vi "Dashboard Main.vi"() -> ()   [LabVIEW 2013]
uses:
  subStates.ctl
  drive safety.ctl
  test controls.ctl
  misc dash data.ctl
  dashboard safety status data.ctl
  <vilib>/event_ctls.llb/lveventtype.ctl
  <vilib>/event_ctls.llb/eventvkey.ctl
  dash error type def.ctl
  <vilib>/Rock Robotics/WPI/DriverStation/WPI_DriverStationDigitalData.ctl
  <vilib>/Utility/config.llb/Write Key (String).vi
  <vilib>/Utility/config.llb/Write Key (I32).vi
  <vilib>/Utility/config.llb/NI_LVConfig.lvlib
panel:
  out "code version":cluster{"code version":string}
  out "connected":string="Connected to robot at IP Address: x.x.x.x"
  in  "Warning No Code":cluster{"Dismiss warning":bool}
  in  "help":bool
  out "no comms":string="NO ROBOT COMMUNICATION"
  in  "no code help":bool
  out "no code":string="NO ROBOT CODE          "
  in  "Warning No Comms":cluster{"Dismiss warning":bool}
  out "Time":string
  out "Drive Safety Data":T1
  out "ip":string="10.0.0.2"
  out "Main Dash SPI":u32
  out "Main Dash IPS":dbl
  out "testmode":bool
  out "lightsense":bool
  out "down":bool
  out "up":bool
  out "unlatched":bool
  out "shooter retracted":bool
  out "Image Message":string="Timeout in Camera Communications"
  in  "Dashboard Tab":T2(tab)
  out "code too slow":bool caption="Robot Code\nRunning too Slow"
  out "Robot Found":bool
  out "BATT":dbl(slide)=12.0 scale=0.0..14.0
  in  "menu":bool
  out "quick data":T4={"Shooter Down"=FALSE, "Shooter Up"=TRUE, "Light Sensor"=FALSE, "Unlatched"=TRUE, "Latched"=TRUE, "State Machine Master"=enum."null", "Dash IPS"=0.0, "Dash mSPI"=0, "Robot IP"="0.0.0.0", "Battery"=16711680, "Code IPS"=0.0, "Code mSPI"=0}
  out "no rate":bool
  out "dist limit":bool
  out "hold":bool
  out "shoot?":bool
  out "Shifter":bool
  out "Vision State":bool
  in  "Camera Settings":T5={"Frame Rate"=30, "Compression"=30, "Size"=1} {"Frame Rate" scale=1.0..30.0; "Size" items=["640x480", "320x240", "160x120"]}
  out "Mode":T6(ring)=enum."Auto Disabled"
  out "Camera IP":string
  in  "DB Camera Config":bool
  out "fps":dbl format="%#.1g"
  out "Mbps":dbl format="%#.1g"
  out "Mbps 2":bool
  out "Distance From Target":dbl
  out "Hot Goal Detected":bool
  out "encoder failure":bool
  out "Directional Failure":bool
  out "TeleOp Elapsed Seconds":dbl
  out "Compressor":u32(colorbox)
  out "info":string="Robot is  in Teleop Disabled"
  out "test disabled":string="Robot is not in Test Mode"
  out "On/Off":bool=TRUE
  out "Full":bool
  out "Charging":bool
  in  "Compressor":bool=TRUE
  out "check settings":string="Check Settings\n\nIf you are trying to test from here,\nchange test mode to dashboard."
  in  "Reset\nManual\nOverrides":bool
  in  "Test \nControls":T7
  out "Test \nIndicators":T8={"Right Distance"=0.0, "Right Rate"=0.0, "Left Distance"=0.0, "Left Rate"=0.0, "Retracted"=TRUE, "Extended"=FALSE, "Shifted Low"=TRUE, "Shifted High"=FALSE, "Unlatched"=TRUE, "Latched"=FALSE, "Directional Issue"=FALSE, "No Rate Read"=FALSE, "Encoder Failure"=FALSE, "At Distance Limit"=FALSE, "Shooter Down"=FALSE, "Shooter Up"=TRUE, "Light Sensor"=FALSE, "Rate"=0.0, "Distance"=0.0, "Right No Rate Read"=FALSE, "Right Encoder Fail"=FALSE, "Left No Rate Read"=FALSE, "LeftEncoder Fail"=FALSE}
  in  "Manual \nOverrides":T9 {"Belts" scale=-1.0..1.0; "Arm" scale=-1.0..1.0; "Drive Train" scale=-1.0..1.0}
  out "timeout error":bool
  out "# of Timeouts":u32
  out "Robot IP\nAddress":string="0.0.0.0"
  out "Solenoid Output":bool[](array[boolean])
  out "8 -- Battery":sgl(graph)
  out "Analog Input":sgl[](array[slide]) scale=0.0..5.0
  out "Drive Encoders":T10
  out "Arm Encoder":cluster{"Distance ":dbl, "Rate":dbl}
  out "Pneumatics":T3
  out "Pickup Arm":T3
  out "Belts":T3
  out "State Machine Master":T3
  out "Drive":T3
  out "Belt Status":u16(ring) items=["Code Control", "Driver Control", "Manual Override"]
  out "Arm Status":u16(ring) items=["Code Control", "Driver Control", "Manual Override"]
  out "Belts":dbl
  out "PWM":cluster{u8, u8}[](array[slide])=[{0, 157}, {0, 157}, {0, 157}, {0, 157}, {0, 157}, {0, 157}, {0, 157}, {0, 157}, {0, 157}, {0, 155}] scale=1.0..255.0
  out "GPIO Output Enable":bool[](array[boolean])
  out "GPIO State":bool[](array[boolean])
  out "Relay":cluster{"Forward":bool[], "Reverse":bool[]}
  out "drive encoder failure":bool
  in  "export stat":bool
  out "Vision mSPI":u32(knob)=100 scale=50.0..200.0
  out "Main mSPI":u32(knob)=20 scale=10.0..40.0
  out "Stats":dbl[][](graph)
  out "cRIO CPU Usage":dbl(knob) scale=0.0..100.0
  out "Vision mSPI":u32
  out "Main mSPI":u32
  out "Main IPS":dbl=50.0
  out "Vision IPS":dbl=10.0
  in  "clear stat":bool
  in  "clear batt":bool
  in  "export batt":bool
  in  "reset":bool
  out "Maximum Voltage":sgl format="%#_gv"
  out "Minimum Voltage":sgl format="%#_gv"
  out "Current Voltage":sgl format="%#_gv"
  out "Battery Stats":sgl(graph)
  in  "Poll Rate (ms)":u32=500
  in  "Listbox":i32(listbox)
  out "Tree":string(tree)
  out "FDC ON":bool
  out "FDC OFF":bool
  in  "Enable Full Driver Control":bool caption="Enables controls with automated functions. Not recommended, since\nthe automated functions were never perfected and are unreliable."
  out "Disable Vision_Off":bool
  out "Disable Vision_On":bool
  in  "Disable Vison After Auto":bool=TRUE caption="After autonomous, vision will be disabled.\nLeave off during practice so multiple \nautonomouses can be run without robot \nreboot being needed. MUST BE ON DURING\nCOMPETITION (DEFAULT)."
  out "Code Version":string
  out "About Speeds":string="Optimal Speeds\n\nMain mSPI = 20\nMain IPS = 50\n\nVision mSPI = 100\nVision IPS = 10\n\nmSPI - miliseconds per iteration\nIPS - iterations per second"
  out "Shoot During\nAuto_Off":bool
  out "Use Hot Goal_Off":bool
  out "2 Ball Auto_Off":bool=TRUE
  out "Shoot During\nAuto_On":bool
  out "Use Hot Goal_On":bool
  out "2 Ball Auto_On":bool
  in  "Shoot During Auto":bool=TRUE caption="When on, shooting sequence will run, \notherwise the robot will just drive forward."
  in  "Use Hot Goal":bool=TRUE caption="Check if the goal is hot when determining \nwhen to shoot, otherwise shoot second cycle."
  in  "2 Ball Auto (Disabled)":bool
  in  "Test Mode":T11(radio)
  in  "Enable":bool
  # "Notification"
  # "!"
  # "C"
  # "No Code"
  # "No robot code has been detected. This means that the code has not \nbegun running yet or there is no code to run.  The code has not\ndeclared to the driver station the code version, so it is assumed \nno code is running."
  # "!"
  # "Warning!"
  # "No robot communication is detected! What to do?\n\n- Is the robot ready and booted? (Blinking RSL)\n- Check robot power.\n- Check various ethernet wire connections on robot and driver station.\n- Check radio power.\n- Robot radio should be on Bridge mode.\n- Check driver station IP address, should be 10.11.24.5, to get it there, simply go to Setup > Choose NIC > Ok (use this espically \n  during competitions). The actual IP should be left alone during competitions since its all special and stuff, so just use that \n  auto-configuring tool.\n- Check diagnostics tab on driver station (bottom of screen, not this) and try to figure it out from there.\n- Contact field personnel if problem persists.\n- Check to make sure that the reason that it's not connecting is not because robots hate you. If this is the case, you should rethink      \n  your ability to drive, be on a robotics team, and ultimately rethink your existence."
  # "Red -  Off, Blue - Charge, Green - Full"
  # "ÜberDashboard 2014"
  # "FRC Team 1124"
  # "ÜberMenu"
  # "Pneumatics"
  # "Home Encoders"
  # "Joystick Control"
  # "Joystick 1"
  # "Joystick 3"
  # "Joystick 2"
  # "Pneumatics"
  # "Arm Encoder"
  # "Drive Train Encoders"
  # "Sensors"
  # "Arm Safety"
  # "Drive Safety"
  # "Manual Override"
  # "Encoders"
  # "Sub-System States"
  # "Belts"
  # "Communications"
  # "Solenoid #1"
  # "1"
  # "8"
  # "Analog #1"
  # "1"
  # "7"
  # "Digital #1"
  # "1"
  # "10"
  # "1"
  # "14"
  # "1"
  # "8"
  # "Main mSPI"
  # "Vision mSPI"
  # "To reset, hold\nreset for 1 \nsecond"
  # "Configure Autonomous\n(Mouse over for info)"
  # "Dash Version 2014_10_09"
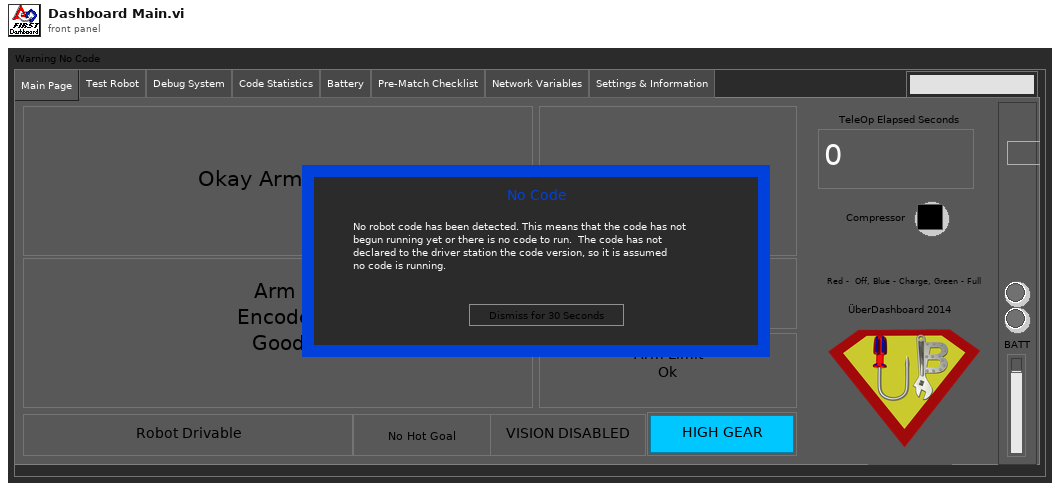
[diagram p1: front panel]
types:
  T1 = typedef "drive safety.ctl" = cluster{"Left - Encoder Failure":bool, "Left - No Rate Read":bool, "Right - Encoder Failure":bool, "Right - No Rate Read":bool}
  T2 = enum32{"Main Page", "Test Robot", "Debug System", "Code Statistics", "Battery", "Pre-Match Checklist", "Network Variables", "Settings & Information"}
  T3 = typedef "subStates.ctl" = enum16{"null", "wait", "driver control", "auto", "manual override", "hold position", "rotate", "pickup", "pass", "recover pass", "load", "goto shoot", "shoot high goal", "shoot low goal", "cancel arm", "cancel shooter", "end", "test"}
  T4 = cluster{"Shooter Down":bool, "Shooter Up":bool, "Light Sensor":bool, "Unlatched":bool, "Latched":bool, "State Machine Master":T3, "Dash IPS":dbl, "Dash mSPI":u32, "Robot IP":string, "Battery":u32, "Code IPS":dbl, "Code mSPI":u32}
  T5 = cluster{"Frame Rate":i32, "Compression":i32, "Size":u16}
  T6 = enum8{"Tele-Op Disabled", "Tele-Op Enabled", "Auto Disabled", "Auto Enabled", "Test Disabled", "Test Enabled", ""}
  T7 = cluster{"Drive Train":bool, "Arm":bool, "Belts":bool, "Home Arm Encoder":bool, "Home Right Drive Encoder":bool, "Home Left Drive Encoder":bool, "Extend Shooter":bool, "Retract Shooter":bool, "Latch":bool, "Unlatch":bool, "Shift High":bool, "Shift Low":bool}
  T8 = cluster{"Right Distance":dbl, "Right Rate":dbl, "Left Distance":dbl, "Left Rate":dbl, "Retracted":bool, "Extended":bool, "Shifted Low":bool, "Shifted High":bool, "Unlatched":bool, "Latched":bool, "Directional Issue":bool, "No Rate Read":bool, "Encoder Failure":bool, "At Distance Limit":bool, "Shooter Down":bool, "Shooter Up":bool, "Light Sensor":bool, "Rate":dbl, "Distance":dbl, "Right No Rate Read":bool, "Right Encoder Fail":bool, "Left No Rate Read":bool, "LeftEncoder Fail":bool}
  T9 = cluster{"Drive Train":dbl, "Arm":dbl, "Belts":dbl}
  T10 = cluster{"Right Rate":dbl, "Left Rate":dbl, "Left Distance":dbl, "Right Distance":dbl}
  T11 = enum32{"Use Dashboard on Driverstation", "Use Programmer's Laptop"}
  T12 = typedef "misc dash data.ctl" = cluster{"Total (%)":dbl, "Vision mSPI":u32, "Main mSPI":u32, "Vision":cluster{"Hot Goal Present?":bool, "distance":dbl}, "Enabled?":bool, "Arm Safety Data":T13, "Drive Safety Data":T1, "TeleOp Elapsed Seconds":dbl}
  T13 = typedef "dashboard safety status data.ctl" = cluster{"At Distance Limit":bool, "No Rate Read":bool, "Encoder Failure":bool, "Encoder Directional Issue":bool}
  T14 = typedef "test controls.ctl" = cluster{"Drive Train":dbl, "Arm":dbl, "Belts":dbl, "Drive Train":bool, "Arm":bool, "Belts":bool, "Home Arm Encoder":bool, "Home Right Drive Encoder":bool, "Home Left Drive Encoder":bool, "Extend Shooter":bool, "Retract Shooter":bool, "Latch":bool, "Unlatch":bool, "Shift High":bool, "Shift Low":bool, "Compressor":bool}
  T15 = typedef "Image Type" = u32
  T16 = typedef "IMAQ Image.ctl" = refnum<image>
  T17 = cluster{"Right Distance":dbl, "Right Rate":dbl, "Left Distance":dbl, "Left Rate":dbl, "Retracted":bool, "Extended":bool, "Shifted Low":bool, "Shifted High":bool, "Unlatched":bool, "Latched":bool, "Directional Issue":bool, "No Rate Read":bool, "Encoder Failure":bool, "At Distance Limit":bool, "Shooter Down":bool, "Shooter Up":bool, "Light Sensor":bool, "Rate":dbl, "Distance":dbl, "Right - No Rate Read":bool, "Right - Encoder Fail":bool, "Left - No Rate Read":bool, "Left - Encoder Fail":bool}
  T18 = typedef "dash error type def.ctl" = cluster{"Timeout Data":cluster{"# of Timeouts":u32, "Time Out Error This Match":bool}, "Can Shoot Safely?":bool}
  T19 = typedef "WPI_DriverStationDigitalData.ctl" = cluster{"Relay Fwd":u8, "Relay Rev":u8, "GPIO":u16, "GPIO_OE":u16, "PWM":cluster{"PWM[0]":u8, "PWM[1]":u8, "PWM[2]":u8, "PWM[3]":u8, "PWM[4]":u8, "PWM[5]":u8, "PWM[6]":u8, "PWM[7]":u8, "PWM[8]":u8, "PWM[9]":u8}}
  T20 = enum8{"Enabled", "Disabled", "Disabled and Grayed Out"}
  T21 = cluster{"Digital Inputs":bool[], "Digital Outputs":bool[]}
  T22 = cluster{"Competition mode":bool, "Robot Link":bool, "Autonomous":bool, "Enabled":bool, "E-Stop":bool, "Simulated":bool, "TestMode":bool, "Docked Window":bool}
  T23 = cluster{"Hot Goal Present?":bool, "distance":dbl}
  T24 = cluster{"# of Timeouts":u32, "Time Out Error This Match":bool}
  T25 = cluster{"Numeric":dbl, "Numeric":dbl, "Numeric":dbl, "Numeric":dbl}
  T26 = typedef "lveventtype.ctl" = enum32{"Null", "Timeout", "Annotation Menu Selection", "Annotation Menu Selection?", "App Instance Close", "App Instance Close?", "Autoscale Range Change", "Bookmark Info Change", "Cell Edit", "Cell Edit?", "Cursor Grab", "Cursor Grab?", "Cursor Menu Selection", "Cursor Menu Selection?", "Cursor Move", "Cursor Release", "Data Change", "Direction Change", "Display State Change", "Drag Ended", "Drag Enter", "Drag Leave", "Drag Over", "Drag Source Update", "Drag Starting", "Drag Starting?", "Drop", "Exec State Change", "Key Down", "Key Down?", "Key Repeat", "Key Repeat?", "Key Up", "Listbox Double Click", "Menu Activation?", "Menu Selection (App)", "Menu Selection? (App)", "Menu Selection (User)", "Mouse Down", "Mouse Down?", "Mouse Enter", "Mouse Leave", "Mouse Move", "Mouse Up", "Mouse Wheel", "NI Security User Change (App)", "Pane Size", "Panel Close", "Panel Close?", "Panel Resize", "Plot Attribute Change", "Scale Range Change", "Shortcut Menu Activation?", "Shortcut Menu Selection (App)", "Shortcut Menu Selection? (App)", "Shortcut Menu Selection (User)", "Tree Double Click", "Tree Drag", "Tree Drag?", "Tree Drop", "Tree Drop?", "Tree Item Close", "Tree Item Close?", "Tree Item Open", "Tree Item Open?", "User Event", "Value Change"}
  T27 = typedef "NI_LVConfig.lvlib/Config Data RefNum.ctl" = refnum<k1>
  T28 = typedef "eventvkey.ctl" = enum16{"ASCII", "Enter", "Return", "Shift", "Ctrl", "Alt", "Cmd", "Opt", "Caps", "NumLock", "Clear", "Break", "Up", "Down", "Left", "Right", "Insert", "Delete", "Home", "End", "PageUp", "PageDown", "Escape", "Help", "Pause", "ScrollLock", "F1", "F2", "F3", "F4", "F5", "F6", "F7", "F8", "F9", "F10", "F11", "F12", "F13", "F14", "F15", "F16", "F17", "F18", "F19", "F20", "F21", "F22", "F23", "F24", "Play", "VolumeUp", "VolumeDown", "Mute", "Two Byte Char"}
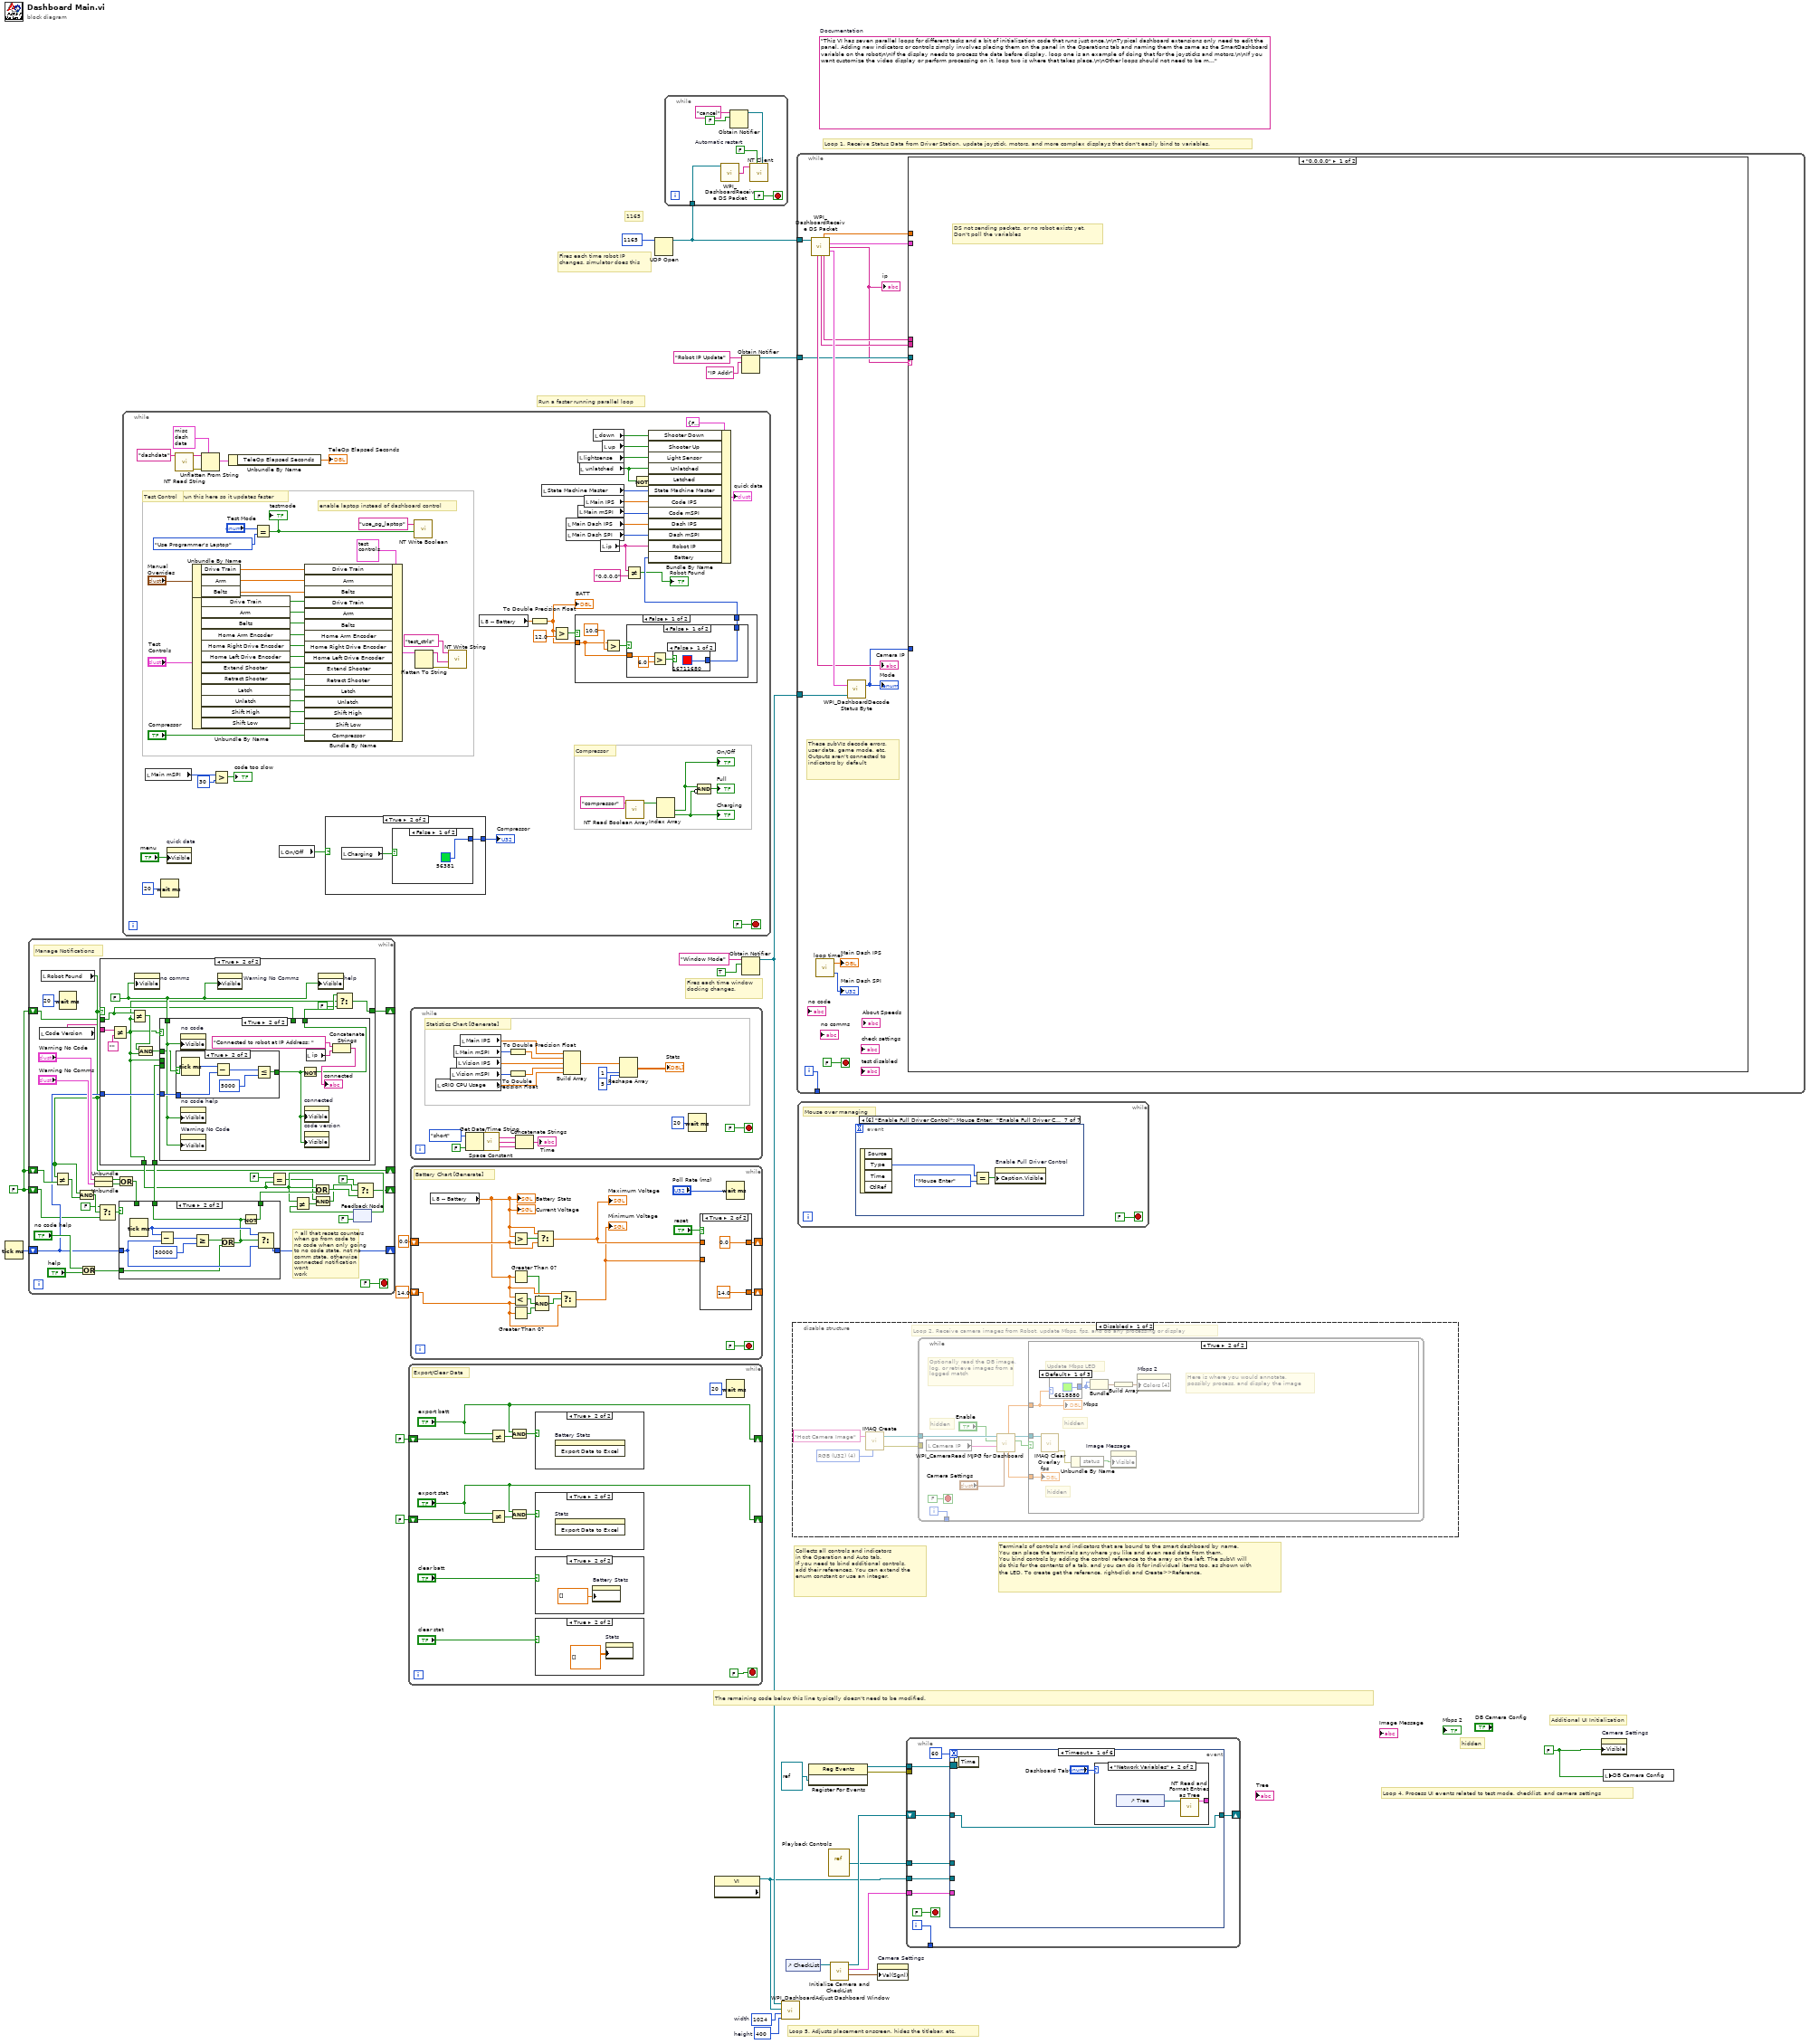
[diagram p0: block diagram]
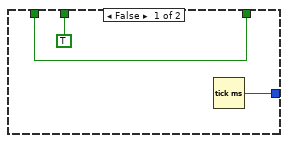
[diagram p7: hidden frame]
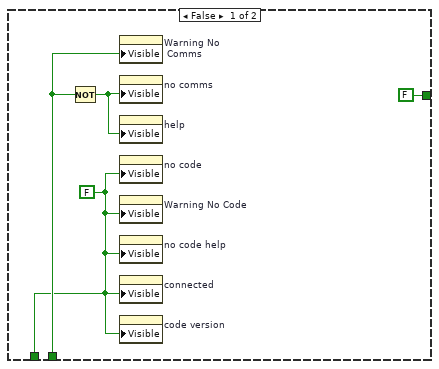
[diagram p8: hidden frame]
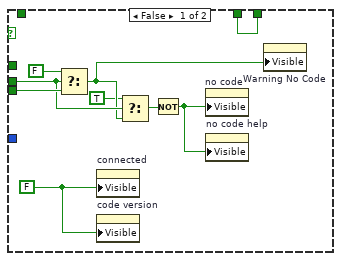
[diagram p9: hidden frame]
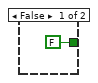
[diagram p10: hidden frame]
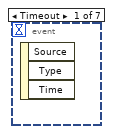
[diagram p11: hidden frame]
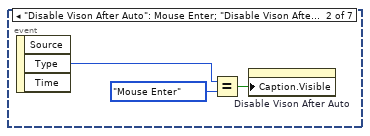
[diagram p12: hidden frame]
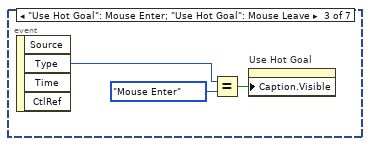
[diagram p13: hidden frame]
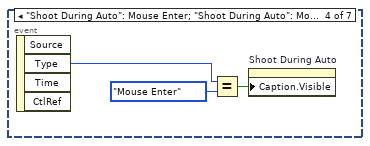
[diagram p14: hidden frame]
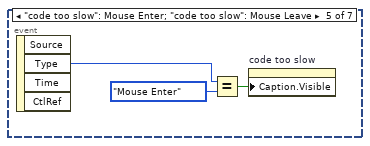
[diagram p15: hidden frame]
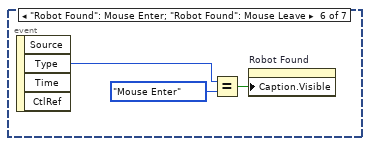
[diagram p16: hidden frame]
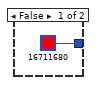
[diagram p17: hidden frame]
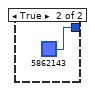
[diagram p18: hidden frame]
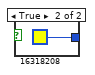
[diagram p19: hidden frame]
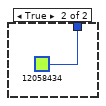
[diagram p20: hidden frame]
diagram:
  w1 = FALSE
  w11 = 400  # height
  w12 = 1024  # width
  w21 = FALSE ("Visible")
  (unwired) "This VI has seven parallel loops for different tasks and a bit of initialization code that runs just once.\n\nTypical dashboard extensions only need to edit the panel. Adding new indicators or controls simply involves placing them on the panel in the Operations tab and naming them the same as the SmartDashboard variable on the robot\n\nIf the display needs to process the data before display, loop one is an example of doing that for the joysticks and motors.\n\nIf you want customize the video display or perform processing on it, loop two is where that takes place.\n\nOther loops should not need to be modified. They are pretty standard, and document the task they perform."  # Documentation
  # "Run a faster running parallel loop"
  # "hidden"
  # "1165"
  # "Loop 4. Process UI events related to test mode, checklist, and camera settings"
  # "Loop 5. Adjusts placement onscreen, hides the titlebar, etc."
  # "Additional UI Initialization"
  # "Fires each time robot IP\nchanges, simulator does this"
  # "Fires each time window\ndocking changes."
  # "Collects all controls and indicators\nin the Operation and Auto tab.\nIf you need to bind additional controls,\nadd their references. You can extend the\nenum constant or use an integer."
  # "The remaining code below this line typically doesn't need to be modified."
  # "Terminals of controls and indicators that are bound to the smart dashboard by name.\nYou can place the terminals anywhere you like and even read data from them.\nYou bind controls by adding the control reference to the array on the left. The subVI will\ndo this for the contents of a tab, and you can do it for individual items too, as shown with\nthe LED. To create get the reference, right-click and Create>>Reference."
  # "Loop 1. Receive Status Data from Driver Station, update joystick, motors, and more complex displays that don't easily bind to variables."
  n1 = Tick Count (ms)() -> (millisecond timer value=w6:u32)
  n2 = while {
    shift-right: [w33] -> _
    shift-left: w1 -> [w43]
    shift-right: [w57] -> _
    shift-left: w6 -> [w46]
    shift-right: [w30] -> _
    shift-left: w1 -> [w47]
    shift-right: [w29] -> _
    shift-left: w1 -> [w28]
    stop <- FALSE stop-if-true
    # "^ all that resets counters\nwhen go from code to\nno code when only going\nto no code state, not no\ncomm state. otherwise \nconnected notification wont\nwork"
    # "Manage Notifications"
    n3 = local read "Code Version"() -> (w27:string)
    n4 = local read "Robot Found"() -> (w30:bool)
    n5 = Not Equal?(x=w30, y=w47) -> (x != y?=w45:bool)
    n6 = Wait (ms)(milliseconds to wait=u32 20) -> ()  [unwired: 1 out]
    n7 = And(x=w30, y=w45) -> (x .and. y?=w44:bool)
    n8 = Or(x="no code help", y="help") -> (x .or. y?=w55:bool)
    n9 = Unbundle("Warning No Code") -> ("Dismiss warning"=w51:bool)
    n10 = Unbundle("Warning No Comms") -> ("Dismiss warning"=w50:bool)
    n11 = Select(t=FALSE, s=w44, f=w43) -> (s? t:f=w42:bool)
    n12 = Or(x=w51, y=w50) -> (x .or. y?=w49:bool)
    n13 = case shown="True" w42 {
      tunnel: w46 -> [_ w69]
      tunnel: [w62 w68] -> w57
      tunnel: [TRUE w64] -> w56
      tunnel: w49 -> [w61 _]
      tunnel: [w61 w67] -> w48
      tunnel: w55 -> [_ w66]
      frame False {
        n14 = Tick Count (ms)() -> (millisecond timer value=w62:u32)
      }
      frame True {
        n15 = Tick Count (ms)() -> (millisecond timer value=w70:u32)
        n16 = Subtract(x=w70, y=w69) -> (x-y=w72:u32)
        n17 = Greater Or Equal?(x=w72, y=u32 30000) -> (x >= y?=w65:bool)
        n18 = Or(x=w65, y=w66) -> (x .or. y?=w64:bool)
        n19 = Not(x=w64) -> (.not. x?=w67:bool)
        n20 = Select(t=w70, s=w64, f=w69) -> (s? t:f=w68:u32)
      }
    }
    n21 = case shown="True" w30 {
      tunnel: w56 -> [w76 w87]
      tunnel: w27 -> [_ w88]
      tunnel: w46 -> [_ w86]
      tunnel: [w74 w77] -> w37
      tunnel: [FALSE w79] -> w29
      tunnel: w28 -> [_ w82]
      frame False {
        w74 = FALSE ("Visible")
        n22 = Not(x=w76) -> (.not. x?=w75:bool)
        n23 = property on="Warning No\n Comms" class="Clust (strict)"("Visible"=w76) -> ()  [unwired: 2 in, 2 out]
        n24 = property on="no comms" class="Str"("Visible"=w75) -> ()  [unwired: 2 in, 2 out]
        n25 = property on="help" class="Bool (strict)"("Visible"=w75) -> ()  [unwired: 2 in, 2 out]
        n26 = property on="no code" class="Str"("Visible"=w74) -> ()  [unwired: 2 in, 2 out]
        n27 = property on="Warning No Code" class="Clust (strict)"("Visible"=w74) -> ()  [unwired: 2 in, 2 out]
        n28 = property on="no code help" class="Bool (strict)"("Visible"=w74) -> ()  [unwired: 2 in, 2 out]
        n29 = property on="connected" class="Str"("Visible"=w74) -> ()  [unwired: 2 in, 2 out]
        n30 = property on="code version" class="Clust (strict)"("Visible"=w74) -> ()  [unwired: 2 in, 2 out]
      }
      frame True {
        w85 = FALSE
        n31 = Not Equal?(x=w88, y="") -> (x != y?=w77:bool)
        n32 = Not Equal?(x=w82, y=w77) -> (x != y?=w84:bool)
        n33 = property on="no comms" class="Str"("Visible"=w85) -> ()  [unwired: 2 in, 2 out]
        n34 = And(x=w84, y=w77) -> (x .and. y?=w81:bool)
        n35 = case shown="True" w77 {
          tunnel: w87 -> [w95 _]
          tunnel: w86 -> [_ w105]
          tunnel: w85 -> [_ w101]
          tunnel: w77 -> [w92 _]
          tunnel: [w89 w98] -> w80
          tunnel: w82 -> [w89 _]
          tunnel: w81 -> [_ w100]
          frame False {
            w96 = FALSE ("Visible")
            n36 = Select(t=FALSE, s=w92, f=w95) -> (s? t:f=w91:bool)
            n37 = property on="connected" class="Str"("Visible"=w96) -> ()  [unwired: 2 in, 2 out]
            n38 = property on="code version" class="Clust (strict)"("Visible"=w96) -> ()  [unwired: 2 in, 2 out]
            n39 = Select(t=TRUE, s=w92, f=w91) -> (s? t:f=w93:bool)
            n40 = Not(x=w93) -> (.not. x?=w97:bool)
            n41 = property on="no code" class="Str"("Visible"=w97) -> ()  [unwired: 2 in, 2 out]
            n42 = property on="no code help" class="Bool (strict)"("Visible"=w97) -> ()  [unwired: 2 in, 2 out]
            n43 = property on="Warning No Code" class="Clust (strict)"("Visible"=w91) -> ()  [unwired: 2 in, 2 out]
          }
          frame True {
            n44 = case shown="True" w100 {
              tunnel: w105 -> [_ w110]
              tunnel: [FALSE w107] -> w99
              frame False {
              }
              frame True {
                n45 = Tick Count (ms)() -> (millisecond timer value=w111:u32)
                n46 = Subtract(x=w111, y=w110) -> (x-y=w108:u32)
                n47 = Less Or Equal?(x=w108, y=u32 5000) -> (x <= y?=w107:bool)
              }
            }
            n48 = property on="no code" class="Str"("Visible"=w101) -> ()  [unwired: 2 in, 2 out]
            n49 = property on="no code help" class="Bool (strict)"("Visible"=w101) -> ()  [unwired: 2 in, 2 out]
            n50 = property on="Warning No Code" class="Clust (strict)"("Visible"=w101) -> ()  [unwired: 2 in, 2 out]
            n51 = Not(x=w99) -> (.not. x?=w98:bool)
            n52 = property on="connected" class="Str"("Visible"=w99) -> ()  [unwired: 2 in, 2 out]
            n53 = property on="code version" class="Clust (strict)"("Visible"=w99) -> ()  [unwired: 2 in, 2 out]
            n54 = local read "ip"() -> (w104:string)
            n55 = Concatenate Strings("Connected to robot at IP Address: ", w104) -> (→"connected":string)
          }
        }
        n56 = property on="Warning No Comms" class="Clust (strict)"("Visible"=w85) -> ()  [unwired: 2 in, 2 out]
        n57 = property on="help" class="Bool (strict)"("Visible"=w85) -> ()  [unwired: 2 in, 2 out]
        n58 = Select(t=w80, s=w77, f=FALSE) -> (s? t:f=w79:bool)
      }
    }
    n59 = Equal?(x=FALSE, y=w37) -> (x = y?=w36:bool)
    n60 = Or(x=w37, y=w48) -> (x .or. y?=w34:bool)
    n61 = feedback-in #1(w37) -> ()
    n62 = feedback #1(FALSE ("code?")) -> (w40:bool)
    n63 = Not Equal?(x=w37, y=w40) -> (x != y?=w39:bool)
    n64 = And(x=w36, y=w39) -> (x .and. y?=w32:bool)
    n65 = Select(t=FALSE, s=w32, f=w34) -> (s? t:f=w33:bool)
  }
  n66 = while {
    stop <- FALSE stop-if-true
    # "Compressor"
    # "run this here so it updates faster"
    # "Test Control"
    # "enable laptop instead of dashboard control"
    n67 = local read "Main mSPI"() -> (w139:u32)
    n68 = Wait (ms)(milliseconds to wait=u32 20) -> ()  [unwired: 1 out]
    n69 = property on="quick data" class="Clust (strict)"("Visible"="menu") -> ()  [unwired: 2 in, 2 out]
    n70 = call <vilib>:"NT Read String.vi"("Name"="dashdata") -> ("error out"=w129:errorcluster, "String"=w130:string)  [unwired: 9 in]
    n71 = Unbundle By Name("Manual \nOverrides") -> ("Drive Train"=w163:dbl, "Arm"=w162:dbl, "Belts"=w161:dbl)
    n72 = Unbundle By Name("Test \nControls") -> ("Drive Train"=w160:bool, "Arm"=w159:bool, "Belts"=w158:bool, "Home Arm Encoder"=w157:bool, "Home Right Drive Encoder"=w156:bool, "Home Left Drive Encoder"=w155:bool, "Extend Shooter"=w154:bool, "Retract Shooter"=w153:bool, "Latch"=w152:bool, "Unlatch"=w151:bool, "Shift High"=w150:bool, "Shift Low"=w149:bool)
    n73 = Unflatten From String(type=T12 {"Total (%)"=0.0, "Vision mSPI"=0, "Main mSPI"=0, "Vision"={"Hot Goal Present?"=FALSE, "distance"=0.0}, "Enabled?"=FALSE, "Arm Safety Data"={"At Distance Limit"=FALSE, "No Rate Read"=FALSE, "Encoder Failure"=FALSE, "Encoder Directional Issue"=FALSE}, "Drive Safety Data"={"Left - Encoder Failure"=FALSE, "Left - No Rate Read"=FALSE, "Right - Encoder Failure"=FALSE, "Right - No Rate Read"=FALSE}, "TeleOp Elapsed Seconds"=0.0} ("Misc Dash Data"), binary string=w130, error in (no error)=w129) -> (value=w127:T12)  [unwired: 2 in, 2 out]
    n74 = Greater?(x=w139, y=u32 30) -> (0:→"code too slow":bool)
    n75 = Unbundle By Name(w127) -> ("TeleOp Elapsed Seconds"=→"TeleOp Elapsed Seconds":dbl)
    n76 = Equal?(x="Test Mode", y=T11."Use Programmer's Laptop") -> (x = y?=w144:bool)
    "testmode" <- w144
    n77 = local read "On/Off"() -> (w113:bool)
    n78 = Bundle By Name(cluster=T14 {"Drive Train"=0.0, "Arm"=0.0, "Belts"=0.0, "Drive Train"=FALSE, "Arm"=FALSE, "Belts"=FALSE, "Home Arm Encoder"=FALSE, "Home Right Drive Encoder"=FALSE, "Home Left Drive Encoder"=FALSE, "Extend Shooter"=FALSE, "Retract Shooter"=FALSE, "Latch"=FALSE, "Unlatch"=FALSE, "Shift High"=FALSE, "Shift Low"=FALSE, "Compressor"=FALSE} ("Test Controls"), "Drive Train"=w163, "Arm"=w162, "Belts"=w161, "Drive Train"=w160, "Arm"=w159, "Belts"=w158, "Home Arm Encoder"=w157, "Home Right Drive Encoder"=w156, "Home Left Drive Encoder"=w155, "Extend Shooter"=w154, "Retract Shooter"=w153, "Latch"=w152, "Unlatch"=w151, "Shift High"=w150, "Shift Low"=w149, "Compressor"="Compressor") -> (w164:T14)
    n79 = case shown="True" w113 {
      tunnel: [u32 16711680 ("Compressor") w180] -> w112
      frame False {
      }
      frame True {
        n80 = local read "Charging"() -> (w179:bool)
        n81 = case shown="False" w179 {
          tunnel: [u32 56381 ("Compressor") u32 5862143 ("Compressor")] -> w180
          frame False {
          }
          frame True {
          }
        }
      }
    }
    "Compressor" <- w112
    n82 = call <vilib>:"NT Write Boolean.vi"("Boolean"=w144, "Name"="use_pg_laptop") -> ()  [unwired: 9 in, 1 out]
    n83 = Flatten To String(anything=w164) -> (data string=w166:string, error out=w167:errorcluster)  [unwired: 3 in, 1 out]
    n84 = call <vilib>:"NT Write String.vi"("error in"=w167, "String"=w166, "Name"="test_ctrls") -> ()  [unwired: 8 in, 1 out]
    n85 = local read "8 -- Battery"() -> (w134:sgl)
    n86 = To Double Precision Float(number=w134) -> (double precision float=w133:dbl)
    "BATT" <- w133
    n87 = local read "State Machine Master"() -> (w173:T3)
    n88 = Greater?(x=w133, y=12.0) -> (0:w135:bool)
    n89 = local read "Main Dash IPS"() -> (w175:dbl)
    n90 = local read "Main Dash SPI"() -> (w174:u32)
    n91 = case shown="False" w135 {
      tunnel: w133 -> [w185 _]
      tunnel: [w183 u32 56369 ("batt status")] -> w132
      frame False {
        n92 = Greater?(x=w185, y=10.0) -> (0:w184:bool)
        n93 = case shown="False" w184 {
          tunnel: w185 -> [w190 _]
          tunnel: [w187 u32 12058434 ("batt status")] -> w183
          frame False {
            n94 = Greater?(x=w190, y=6.0) -> (0:w188:bool)
            n95 = case shown="False" w188 {
              tunnel: [u32 16711680 ("batt status") u32 16318208 ("batt status")] -> w187
              frame False {
              }
              frame True {
              }
            }
          }
          frame True {
          }
        }
      }
      frame True {
      }
    }
    n96 = local read "Main mSPI"() -> (w115:u32)
    n97 = local read "lightsense"() -> (w170:bool)
    n98 = local read "unlatched"() -> (w168:bool)
    n99 = local read "Main IPS"() -> (w116:dbl)
    n100 = local read "down"() -> (w172:bool)
    n101 = local read "ip"() -> (w141:string)
    n102 = local read "up"() -> (w171:bool)
    n103 = Not Equal?(x=w141, y="0.0.0.0") -> (x != y?=→"Robot Found":bool)
    n104 = call <vilib>:"NT Read Boolean Array.vi"("Name"="compressor") -> ("Boolean Array"=w122:bool[])  [unwired: 9 in, 1 out]
    n105 = Not(x=w168) -> (.not. x?=w169:bool)
    n106 = Bundle By Name(cluster=T4 {"Shooter Down"=FALSE, "Shooter Up"=FALSE, "Light Sensor"=FALSE, "Unlatched"=FALSE, "Latched"=TRUE, "State Machine Master"=enum."null", "Dash IPS"=50.0, "Dash mSPI"=20, "Robot IP"="10.0.0.2", "Battery"=16711680, "Code IPS"=50.0, "Code mSPI"=20} ("quick data"), "Shooter Down"=w172, "Shooter Up"=w171, "Light Sensor"=w170, "Unlatched"=w168, "Latched"=w169, "State Machine Master"=w173, "Code IPS"=w116, "Code mSPI"=w115, "Dash IPS"=w175, "Dash mSPI"=w174, "Robot IP"=w141, "Battery"=w132) -> (→"quick data":T4)
    n107 = Index Array(array=w122) -> (element #1=w120:bool, element #2=w119:bool)  [unwired: 2 in]
    "Charging" <- w119
    "On/Off" <- w120
    n108 = Compound Arithmetic op=AND(w120, invert w119) -> (→"Full":bool)
  }
  n109 = while {
    shift-right: ["export batt"] -> _
    shift-left: FALSE ("export batt") -> [w204]
    shift-right: ["export stat"] -> _
    shift-left: FALSE ("export batt") -> [w200]
    stop <- FALSE stop-if-true
    # "Export/Clear Data"
    n110 = Not Equal?(x="export batt", y=w204) -> (x != y?=w205:bool)
    n111 = Not Equal?(x="export stat", y=w200) -> (x != y?=w199:bool)
    n112 = And(x="export batt", y=w205) -> (x .and. y?=w206:bool)
    n113 = And(x="export stat", y=w199) -> (x .and. y?=w198:bool)
    n114 = case shown="True" w206 {
      frame False {
      }
      frame True {
        n115 = invoke on="Battery Stats" class="WFChart (strict)" method="Export Data to Excel"() -> ()  [unwired: 3 in, 3 out]
      }
    }
    n116 = case shown="True" w198 {
      frame False {
      }
      frame True {
        n117 = invoke on="Stats" class="WFChart (strict)" method="Export Data to Excel"() -> ()  [unwired: 3 in, 3 out]
      }
    }
    n118 = case shown="True" "clear batt" {
      frame False {
      }
      frame True {
        n119 = property on="Battery Stats" class="WFChart (strict)"("History Data"=sgl[] []) -> ()  [unwired: 2 in, 2 out]
      }
    }
    n120 = case shown="True" "clear stat" {
      frame False {
      }
      frame True {
        n121 = property on="Stats" class="WFChart (strict)"("History Data"=dbl[][] []) -> ()  [unwired: 2 in, 2 out]
      }
    }
    n122 = Wait (ms)(milliseconds to wait=u32 20) -> ()  [unwired: 1 out]
  }
  n123 = while {
    stop <- FALSE stop-if-true
    # "Statistics Chart [Generate]"
    n124 = local read "cRIO CPU Usage"() -> (w226:dbl)
    n125 = local read "Vision mSPI"() -> (w225:u32)
    n126 = local read "Main mSPI"() -> (w222:u32)
    n127 = local read "Vision IPS"() -> (w221:dbl)
    n128 = local read "Main IPS"() -> (w227:dbl)
    n129 = Get Date/Time String(date format (0)=enum16{"short", "long", "abbreviated"}."short", want seconds? (F)=FALSE) -> (date string=w210:string, time string=w211:string)  [unwired: 1 in]
    n130 = call <vilib>:"Space Constant.vi"() -> ("String"=w212:string)
    n131 = To Double Precision Float(number=w222) -> (double precision float=w223:dbl)
    n132 = To Double Precision Float(number=w225) -> (double precision float=w224:dbl)
    n133 = Concatenate Strings(w210, w212, w211) -> (→"Time":string)
    n134 = Build Array(w227, w223, w221, w224, w226) -> (w219:dbl[])
    n135 = Reshape Array(w219, 1 ("dimension size"), 5 ("dimension size")) -> (→"Stats":dbl[][])
    n136 = Wait (ms)(milliseconds to wait=u32 20) -> ()  [unwired: 1 out]
  }
  n137 = while {
    shift-right: [w235] -> _
    shift-left: sgl 0.0 ("Current Voltage") -> [w239]
    shift-right: [w234] -> _
    shift-left: sgl 14.0 ("Current Voltage") -> [w230]
    stop <- FALSE stop-if-true
    # "Battery Chart [Generate]"
    n138 = local read "8 -- Battery"() -> (w229:sgl)
    "Battery Stats" <- w229
    "Current Voltage" <- w229
    n139 = Greater?(x=w229, y=w239) -> (0:w240:bool)
    n140 = Greater Than 0?(x=w229) -> (x > 0?=w228:bool)
    n141 = Less?(x=w229, y=w230) -> (x < y?=w233:bool)
    n142 = Greater Than 0?(x=w230) -> (x > 0?=w232:bool)
    n143 = Compound Arithmetic op=AND(w228, w233, w232) -> (w231:bool)
    n144 = Select(t=w229, s=w240, f=w239) -> (s? t:f=w238:sgl)
    "Maximum Voltage" <- w238
    n145 = Select(t=w229, s=w231, f=w230) -> (s? t:f=w237:sgl)
    "Minimum Voltage" <- w237
    n146 = case shown="True" "reset" {
      tunnel: w238 -> [w244 _]
      tunnel: w237 -> [w243 _]
      tunnel: [w244 sgl 0.0 ("Current Voltage")] -> w235
      tunnel: [w243 sgl 14.0 ("Current Voltage")] -> w234
      frame False {
      }
      frame True {
      }
    }
    n147 = Wait (ms)(milliseconds to wait="Poll Rate (ms)") -> ()  [unwired: 1 out]
  }
  n148 = UDP Open(11:u16 1165 ("port")) -> (port=w8:refnum<k16>)  [unwired: 2 in, 4 out]
  n149 = while {
    tunnel: w8 -> [w248]
    stop <- FALSE stop-if-true
    w253 = FALSE  # Automatic restart
    n150 = call <vilib>:"WPI_DashboardReceive DS Packet.vi"("Recv Socket"=w248) -> ("Robot IP Address"=w249:string)  [unwired: 1 in, 13 out]
    n151 = Obtain Notifier(name (unnamed)="cancel", notification data type=FALSE) -> (notifier out=w250:refnum<notifier>)  [unwired: 2 in, 2 out]
    n152 = call <vilib>:"NT Client.vi"("Cancel Ref"=w250, "Automatic restart"=w253, "Server IP Address"=w249) -> ()  [unwired: 9 in]
  }
  n153 = property class="VI" props=["Front Panel.Closeable"]() -> (reference out=w9:refnum<vi>)  [unwired: 2 in, 2 out]
  n154 = Obtain Notifier(name (unnamed)="Robot IP Update", notification data type="IP Addr" ("name (unnamed)")) -> (notifier out=w23:refnum<notifier>)  [unwired: 2 in, 2 out]
  n155 = Obtain Notifier(name (unnamed)="Window Mode", notification data type=TRUE) -> (notifier out=w20:refnum<notifier>)  [unwired: 2 in, 2 out]
  n156 = call <vilib>:"WPI_DashboardAdjust Dashboard Window.vi"("height"=w11, "width"=w12, "reference in"=w9, "Notifier in"=w20) -> ()  [unwired: 8 in]
  n157 = control-ref of="CheckList"() -> (w10:refnum<vi>)
  n158 = disable-structure shown="Disabled" {
    frame Disabled {
      w257 = T15 4 items=["Grayscale (U8)", "Grayscale (I16)", "Grayscale (SGL)", "Complex (CSG)", "RGB (U32)", "HSL (U32)", "RGB (U64)"] ("Image Type")
      # "Loop 2. Receive camera images from Robot, update Mbps, fps, and do any processing or display"
      n159 = call "IMAQ Create"("Image Name"="Host Camera Image", "Image Type"=w257) -> ("New Image"=w255:T16, "error out"=w254:errorcluster)  [unwired: 2 in, 1 out]
      n160 = while {
        tunnel: w255 -> [w265]
        tunnel: w254 -> [_]
        tunnel: [w266] -> _
        i -> [w266]
        stop <- FALSE stop-if-true
        # "hidden"
        # "Optionally read the DB image,\nlog, or retrieve images from a\nlogged match"
        n161 = local read "Camera IP"() -> (w258:string)
        n162 = call <vilib>:"WPI_CameraRead MJPG for Dashboard.vi"("Camera Settings"="Camera Settings", "Camera IP"=w258, "Enable"="Enable", "Refnum in"=w265) -> ("Active"=w262:bool, "Refnum out"=w264:T16, "FPS"=w261:dbl, "Bandwidth (Mbps)"=w260:dbl)  [unwired: 4 in]
        n163 = case shown="True" w262 {
          tunnel: w264 -> [_ w272]
          tunnel: w260 -> [_ w271]
          tunnel: w261 -> [_ w269]
          frame False {
            # "Sleep for 500ms"
            n164 = Wait Until Next ms Multiple(millisecond multiple=u32 500) -> ()  [unwired: 1 out]
          }
          frame True {
            # "hidden"
            # "hidden"
            # "Here is where you would annotate,\npossibly process, and display the image"
            # "Update Mbps LED"
            n165 = call "IMAQ Clear Overlay"("Image"=w272) -> ("error out"=w276:errorcluster, "Image Out"=w270:T16)  [unwired: 2 in, 7 out]
            n166 = case shown="Default" w271 {
              tunnel: [u32 6618880 ("Color Box") u32 16776722 ("Color Box") u32 16716800 ("Color Box")] -> w273
              frame Default {
              }
              frame 4, 5 {
              }
              frame 6.. {
              }
            }
            n167 = Unbundle By Name(w276) -> ("status"=w277:bool)
            n168 = Bundle("Color Box"=w273, "Color Box"=w273) -> (w275:cluster{"Color Box":u32, "Color Box":u32})  [unwired: 1 out]
            n169 = property on="Image Message" class="Str"("Visible"=w277) -> ()  [unwired: 2 in, 2 out]
            n170 = Build Array(w275) -> (w274:cluster{"Color Box":u32, "Color Box":u32}[])
            n171 = property on="Mbps 2" class="Bool (strict)"("Colors [4]"=w274) -> ()  [unwired: 2 in, 2 out]
            "Mbps" <- w271
            "fps" <- w269
          }
        }
      }
    }
    frame Enabled {
    }
  }
  n172 = while {
    tunnel: w8 -> [w293]
    tunnel: w23 -> [w289]
    tunnel: w20 -> [w292]
    tunnel: [w290] -> _
    i -> [w290]
    stop <- FALSE stop-if-true
    # "These subVIs decode errors, user data, game mode, etc.\nOutputs aren't connected to indicators by default"
    n173 = call <vilib>:"WPI_DashboardReceive DS Packet.vi"("Recv Socket"=w293) -> ("Battery"=w285:sgl, "Driver Station"=w286:T21, "Robot IP Address"=w281:string, "Status"=w294:T22, "Camera IP Address"=→"Camera IP":string, "Low Priority User Data"=w288:string, "High Priority User Data"=w287:string)  [unwired: 1 in, 7 out]
    "ip" <- w281
    n174 = call "loop timer.vi"() -> ("IPS"=→"Main Dash IPS":dbl, "SPI"=→"Main Dash SPI":u32)  [unwired: 1 in]
    n175 = call <vilib>:"WPI_DashboardDecode Status Byte.vi"("Window Mode Notifier"=w292, "Status"=w294) -> ("Mode"=w284:T6)  [unwired: 1 out]
    "Mode" <- w284
    n176 = case shown="\"0.0.0.0\"" w281 {
      selector: w281 -> [_ w332]
      tunnel: w289 -> [_ w457]
      tunnel: w288 -> [_ _]
      tunnel: w287 -> [_ _]
      tunnel: w286 -> [_ _]
      tunnel: w285 -> [_ w435]
      tunnel: w284 -> [_ w371]
      frame "0.0.0.0" {
        # "DS not sending packets, or no robot exists yet.\nDon't poll the variables"
      }
      frame Default {
        w335 = inf ("x")
        w334 = 0.0 ("t")
        # "DS sent a packet. use any data it\nprovided, poll others and update\ndisplays that don'teasily bind\nusing names"
        # "Autonomous Configuration"
        # "States"
        # "Full Driver Control"
        # "Check Code Version"
        # "Notify Drivers of Encoder Failure"
        # "Hidden, not in use"
        # "Accumulate Test Indication Data"
        # "Test Visuals and Reinits"
        # "Misc Data"
        # "Timeouts and Safeshoot"
        # "Encoders"
        # "Motors"
        # "Digital, Analog, and Solenoids"
        # "Notify NT\nBind loop"
        n177 = local read "testmode"() -> (w340:bool)
        n178 = Send Notification(notification=w332, notifier=w457) -> ()  [unwired: 1 in, 2 out]
        n179 = case shown="True" "Reset\nManual\nOverrides" {
          frame False {
          }
          frame True {
            n180 = invoke on="Manual \nOverrides" class="Clust (strict)" method="Reinit To Default"() -> ()  [unwired: 3 in, 3 out]
          }
        }
        n181 = Format Into String(initial string="Robot is in ", w371) -> (resulting string=→"info":string)  [unwired: 2 in, 1 out]
        n182 = Equal?(x=w371, y=T6."Test Enabled") -> (x = y?=w341:bool)
        n183 = local read "Drive Safety Data"() -> (w302:T1)
        n184 = Compound Arithmetic op=AND(w341, invert w340) -> (w343:bool)
        n185 = local read "Drive Encoders"() -> (w348:T10)
        n186 = local read "shooter retracted"() -> (w366:bool)
        n187 = local read "Shifter"() -> (w364:bool)
        n188 = local read "unlatched"() -> (w360:bool)
        n189 = local read "Directional Failure"() -> (w373:bool)
        n190 = local read "no rate"() -> (w374:bool)
        n191 = local read "encoder failure"() -> (w370:bool)
        n192 = local read "dist limit"() -> (w369:bool)
        n193 = local read "down"() -> (w354:bool)
        n194 = local read "up"() -> (w353:bool)
        n195 = local read "lightsense"() -> (w350:bool)
        n196 = local read "Arm Encoder"() -> (w377:cluster{"Distance ":dbl, "Rate":dbl})
        n197 = call <vilib>:"NT Read Numeric Array.vi"("Name"="analog") -> ("Numeric Array"=w437:dbl[])  [unwired: 9 in, 1 out]
        n198 = case shown="False" w343 {
          tunnel: [T20."Disabled and Grayed Out" ("Disabled") T20."Enabled" ("Disabled")] -> w331
          frame False {
          }
          frame True {
          }
        }
        n199 = And(x=w341, y=w340) -> (x .and. y?=w342:bool)
        n200 = Build Array("Disable Vison After Auto", "2 Ball Auto (Disabled)", "Use Hot Goal", "Shoot During Auto") -> (w313:bool[])
        n201 = To Single Precision Float(number=w437) -> (single precision float=→"Analog Input":sgl[])
        n202 = property on="check settings" class="Str"("Visible"=w342) -> ()  [unwired: 2 in, 2 out]
        n203 = Not(x="Disable Vison After Auto") -> (.not. x?=→"Disable Vision_Off":bool)
        n204 = Not(x="2 Ball Auto (Disabled)") -> (.not. x?=→"2 Ball Auto_Off":bool)
        n205 = Not(x="Use Hot Goal") -> (.not. x?=→"Use Hot Goal_Off":bool)
        n206 = Not(x="Shoot During Auto") -> (.not. x?=→"Shoot During\nAuto_Off":bool)
        n207 = disable-structure shown="Enabled" {
          disable-tunnel: [_ T19 {"Relay Fwd"=0, "Relay Rev"=0, "GPIO"=0, "GPIO_OE"=0, "PWM"={"PWM[0]"=0, "PWM[1]"=0, "PWM[2]"=0, "PWM[3]"=0, "PWM[4]"=0, "PWM[5]"=0, "PWM[6]"=0, "PWM[7]"=0, "PWM[8]"=0, "PWM[9]"=0}} ("DigitalModule")] -> w383
          frame Disabled {
            (unwired) T19[] [] ("array")
          }
          frame Enabled {
          }
        }
        n208 = Not(x=w343) -> (.not. x?=w379:bool)
        n209 = Unbundle By Name(w302) -> ("Left - Encoder Failure"=w322:bool, "Left - No Rate Read"=w328:bool, "Right - Encoder Failure"=w327:bool, "Right - No Rate Read"=w326:bool)
        n210 = property on="test disabled" class="Str"("Visible"=w379) -> ()  [unwired: 2 in, 2 out]
        n211 = property on="info" class="Str"("Visible"=w379) -> ()  [unwired: 2 in, 2 out]
        n212 = call <vilib>:"NT Write Boolean Array.vi"("Boolean Array"=w313, "Name"="auto_config") -> ()  [unwired: 9 in, 1 out]
        n213 = Unbundle By Name(w348) -> ("Right Distance"=w349:dbl, "Right Rate"=w347:dbl, "Left Distance"=w346:dbl, "Left Rate"=w345:dbl)
        n214 = Unbundle By Name(w377) -> ("Rate"=w376:dbl, "Distance"=w375:dbl)
        n215 = call <vilib>:"NT Read String.vi"("Name"="dio") -> ("error out"=w425:errorcluster, "String"=w426:string)  [unwired: 9 in]
        n216 = Not(x=w366) -> (.not. x?=w365:bool)
        n217 = Not(x=w364) -> (.not. x?=w361:bool)
        n218 = Not(x=w360) -> (.not. x?=w359:bool)
        n219 = property on="Test \nControls" class="Clust (strict)"("DisabledEnum"=w331) -> ()  [unwired: 2 in, 2 out]
        n220 = property on="Test \nIndicators" class="Clust (strict)"("DisabledEnum"=w331) -> ()  [unwired: 2 in, 2 out]
        n221 = property on="Manual \nOverrides" class="Clust (strict)"("DisabledEnum"=w331) -> ()  [unwired: 2 in, 2 out]
        n222 = property on="Reset\nManual\nOverrides" class="Bool (strict)"("DisabledEnum"=w331) -> ()  [unwired: 2 in, 2 out]
        n223 = property on="On/Off" class="Bool (strict)"("DisabledEnum"=w331) -> ()  [unwired: 2 in, 2 out]
        n224 = property on="Full" class="Bool (strict)"("DisabledEnum"=w331) -> ()  [unwired: 2 in, 2 out]
        n225 = property on="Charging" class="Bool (strict)"("DisabledEnum"=w331) -> ()  [unwired: 2 in, 2 out]
        n226 = property on="Compressor" class="Bool (strict)"("DisabledEnum"=w331) -> ()  [unwired: 2 in, 2 out]
        n227 = Unflatten From String(type=w383, binary string=w426, error in (no error)=w425) -> (value=w382:T19)  [unwired: 2 in, 2 out]
        n228 = Bundle By Name(cluster=T17 {"Right Distance"=0.0, "Right Rate"=0.0, "Left Distance"=0.0, "Left Rate"=0.0, "Retracted"=TRUE, "Extended"=FALSE, "Shifted Low"=TRUE, "Shifted High"=FALSE, "Unlatched"=TRUE, "Latched"=FALSE, "Directional Issue"=FALSE, "No Rate Read"=FALSE, "Encoder Failure"=FALSE, "At Distance Limit"=FALSE, "Shooter Down"=FALSE, "Shooter Up"=TRUE, "Light Sensor"=FALSE, "Rate"=0.0, "Distance"=0.0, "Right - No Rate Read"=FALSE, "Right - Encoder Fail"=FALSE, "Left - No Rate Read"=FALSE, "Left - Encoder Fail"=FALSE} ("Test \nIndicators"), "Right Distance"=w349, "Right Rate"=w347, "Left Distance"=w346, "Left Rate"=w345, "Retracted"=w366, "Extended"=w365, "Shifted Low"=w364, "Shifted High"=w361, "Unlatched"=w360, "Latched"=w359, "Directional Issue"=w373, "No Rate Read"=w374, "Encoder Failure"=w370, "At Distance Limit"=w369, "Shooter Down"=w354, "Shooter Up"=w353, "Light Sensor"=w350, "Rate"=w376, "Distance"=w375, "Left - Encoder Fail"=w322, "Left - No Rate Read"=w328, "Right - Encoder Fail"=w327, "Right - No Rate Read"=w326) -> (→"Test \nIndicators":T17)
        n229 = disable-structure shown="Enabled" {
          disable-tunnel: w382 -> [_ w460]
          disable-tunnel: [_ w460] -> w381
          frame Disabled {
            n230 = Index Array() -> ()  [unwired: 2 in, 1 out]
          }
          frame Enabled {
          }
        }
        n231 = call <vilib>:"NT Read Number.vi"("Name"="solenoids") -> ("Numeric"=w423:dbl)  [unwired: 9 in, 1 out]
        n232 = call "Parse Digital Module.vi"("DigitalModule"=w381) -> ("GPIO Output Enable"=→"GPIO Output Enable":bool[], "GPIO State"=w316:bool[], "PWM"=→"PWM":cluster{u8, u8}[], "Relay"=→"Relay":cluster{"Forward":bool[], "Reverse":bool[]})  [unwired: 7 in]
        n233 = To Unsigned Byte Integer(number=w423) -> (unsigned 8bit integer=w422:u8)
        n234 = Not(x=w316) -> (.not. x?=w315:bool[])
        "GPIO State" <- w315
        n235 = Not(x="Enable Full Driver Control") -> (.not. x?=→"FDC OFF":bool)
        n236 = call <vilib>:"NT Read String.vi"("Name"="dashdata") -> ("error out"=w409:errorcluster, "String"=w408:string)  [unwired: 9 in]
        n237 = Number To Boolean Array(number=w422) -> (Boolean array=w421:bool[])
        "Solenoid Output" <- w421
        n238 = Unflatten From String(type=T12 {"Total (%)"=0.0, "Vision mSPI"=0, "Main mSPI"=0, "Vision"={"Hot Goal Present?"=FALSE, "distance"=0.0}, "Enabled?"=FALSE, "Arm Safety Data"={"At Distance Limit"=FALSE, "No Rate Read"=FALSE, "Encoder Failure"=FALSE, "Encoder Directional Issue"=FALSE}, "Drive Safety Data"={"Left - Encoder Failure"=FALSE, "Left - No Rate Read"=FALSE, "Right - Encoder Failure"=FALSE, "Right - No Rate Read"=FALSE}, "TeleOp Elapsed Seconds"=0.0} ("Misc Dash Data"), binary string=w408, error in (no error)=w409) -> (value=w406:T12)  [unwired: 2 in, 2 out]
        n239 = call <vilib>:"SD Write Boolean.vi"("Boolean"="Enable Full Driver Control", "Name"="fdc") -> ()  [unwired: 8 in, 2 out]
        n240 = local read "Drive Safety Data"() -> (w301:T1)
        n241 = Unbundle By Name(w406) -> ("Drive Safety Data"=→"Drive Safety Data":T1, "Arm Safety Data"=w402:T13, "Total (%)"=→"cRIO CPU Usage":dbl, "Vision mSPI"=w400:u32, "Main mSPI"=w401:u32, "Vision"=w405:T23, "Enabled?"=→"Vision State":bool)
        "Vision mSPI" <- w400
        "Main mSPI" <- w401
        n242 = Index Array(array=w421, index #1=5 ("index"), index #2=2 ("index"), index #3=1 ("index")) -> (element #1=→"Shifter":bool, element #2=→"shooter retracted":bool, element #3=→"unlatched":bool)
        n243 = Index Array(array=w315, index #1=6 ("index"), index #2=7 ("index"), index #3=11 ("index")) -> (element #1=→"up":bool, element #2=→"down":bool, element #3=→"lightsense":bool)
        n244 = Unbundle(w301) -> ("Left - Encoder Failure"=w321:bool, "Left - No Rate Read"=w320:bool, "Right - Encoder Failure"=w319:bool, "Right - No Rate Read"=w318:bool)
        n245 = call <vilib>:"NT Read String.vi"("Name"="errors") -> ("error out"=w415:errorcluster, "String"=w414:string)  [unwired: 9 in]
        n246 = Unbundle By Name(w402) -> ("Encoder Failure"=→"encoder failure":bool, "Encoder Directional Issue"=→"Directional Failure":bool, "At Distance Limit"=→"dist limit":bool, "No Rate Read"=→"no rate":bool)
        n247 = Compound Arithmetic op=OR(w321, w320, w319, w318) -> (→"drive encoder failure":bool)
        n248 = call <vilib>:"NT Read String.vi"("Name"="code_rev") -> ("String"=w299:string)  [unwired: 9 in, 1 out]
        "Code Version" <- w299
        n249 = Unflatten From String(type=T18 {"Timeout Data"={"# of Timeouts"=0, "Time Out Error This Match"=FALSE}, "Can Shoot Safely?"=FALSE} ("Errors"), binary string=w414, error in (no error)=w415) -> (value=w412:T18)  [unwired: 2 in, 2 out]
        n250 = call <vilib>:"NT Read Numeric Array.vi"("Name"="subsystem_states") -> ("Numeric Array"=w433:dbl[])  [unwired: 9 in, 1 out]
        n251 = Unbundle By Name(w405) -> ("distance"=→"Distance From Target":dbl, "Hot Goal Present?"=→"Hot Goal Detected":bool)
        n252 = Unbundle By Name(w412) -> ("Timeout Data"=w410:T24, "Can Shoot Safely?"=→"shoot?":bool)
        n253 = To Double Precision Float(number=w400) -> (double precision float=w444:dbl)
        n254 = To Double Precision Float(number=w401) -> (double precision float=w449:dbl)
        n255 = To Unsigned Word Integer(number=w433) -> (unsigned 16bit integer=w432:u16[])
        n256 = call <vilib>:"NT Read Numeric Array.vi"("Name"="encoders") -> ("Numeric Array"=w399:dbl[])  [unwired: 9 in, 1 out]
        n257 = Reciprocal(x=w444) -> (1/x=w445:dbl)
        n258 = Reciprocal(x=w449) -> (1/x=w448:dbl)
        n259 = Index Array(array=w432) -> (element #1=w420:u16, element #2=→"State Machine Master":u16, element #3=w429:u16, element #4=w430:u16, element #5=→"Pneumatics":u16)  [unwired: 5 in]
        "Drive" <- w420
        "Belts" <- w429
        "Pickup Arm" <- w430
        n260 = Concatenate Strings("Connected to Robot!\nCode Version: ", w299) -> (w297:string)
        n261 = Index Array(array=w399) -> (element #1=w398:dbl, element #2=w397:dbl, element #3=w396:dbl, element #4=w395:dbl, element #5=w394:dbl, element #6=w393:dbl)  [unwired: 6 in]
        n262 = case shown="0, Default" w429 {
          tunnel: [w464 w465 w466] -> w442
          frame 0, Default {
            w464 = u16 0 items=["Code Control", "Driver Control", "Manual Override"] ("Arm Status")
          }
          frame 2 {
            w465 = u16 1 items=["Code Control", "Driver Control", "Manual Override"] ("Arm Status")
          }
          frame 4 {
            w466 = u16 2 items=["Code Control", "Driver Control", "Manual Override"] ("Arm Status")
          }
        }
        "Belt Status" <- w442
        n263 = case shown="0, Default" w430 {
          tunnel: [w467 w468 w469] -> w441
          frame 0, Default {
            w467 = u16 0 items=["Code Control", "Driver Control", "Manual Override"] ("Arm Status")
          }
          frame 2 {
            w468 = u16 1 items=["Code Control", "Driver Control", "Manual Override"] ("Arm Status")
          }
          frame 4 {
            w469 = u16 2 items=["Code Control", "Driver Control", "Manual Override"] ("Arm Status")
          }
        }
        "Arm Status" <- w441
        n264 = Multiply(x=w445, y=1000.0) -> (x*y=w333:dbl)
        n265 = Multiply(x=w448, y=1000.0) -> (x*y=w338:dbl)
        n266 = Equal?(x=subStates."hold position" ("Drive"), y=w420) -> (x = y?=→"hold":bool)
        n267 = Unbundle By Name(w410) -> ("# of Timeouts"=→"# of Timeouts":u32, "Time Out Error This Match"=→"timeout error":bool)
        n268 = Bundle(cluster=cluster{"code version":string} {"code version"="Connected to Robot!\nCode Version: 2014_10_06_v1_BASH"} ("code version"), "code version"=w297) -> (→"code version":cluster{"code version":string})
        n269 = Equal?(x=w335, y=w333) -> (x = y?=w387:bool)
        n270 = Equal?(x=w335, y=w338) -> (x = y?=w339:bool)
        n271 = local read "Vision mSPI"() -> (→"Vision mSPI":u32)
        n272 = local read "Main mSPI"() -> (→"Main mSPI":u32)
        n273 = call <vilib>:"NT Read Number.vi"("Name"="belts") -> ("Numeric"=→"Belts":dbl)  [unwired: 9 in, 1 out]
        n274 = Bundle("Numeric"=w397, "Numeric"=w395, "Numeric"=w396, "Numeric"=w398) -> (→"Drive Encoders":T25)  [unwired: 1 in]
        n275 = Bundle("Numeric"=w394, "Numeric"=w393) -> (→"Arm Encoder":cluster{"Numeric":dbl, "Numeric":dbl})  [unwired: 1 in]
        n276 = Select(t=w334, s=w387, f=w333) -> (s? t:f=→"Vision IPS":dbl)
        n277 = Select(t=w334, s=w339, f=w338) -> (s? t:f=→"Main IPS":dbl)
        "8 -- Battery" <- w435
        "Robot IP\nAddress" <- w332
        "2 Ball Auto_On" <- "2 Ball Auto (Disabled)"
        "Use Hot Goal_On" <- "Use Hot Goal"
        "Shoot During\nAuto_On" <- "Shoot During Auto"
        "Disable Vision_On" <- "Disable Vison After Auto"
        "FDC ON" <- "Enable Full Driver Control"
      }
    }
  }
  n278 = while {
    stop <- FALSE stop-if-true
    # "Mouse over managing"
    n279 = event shown="[6] \"Enable Full Driver Control\": Mouse Enter;  \"Enable Full Driver Control\": Mouse Leave" {
      selector: _ -> [_ _ _ _ _ _ _]
      dyn-events: _ -> [_ _ _ _ _ _ _]
      timeout: _ -> [_ _ _ _ _ _ _]
      event Timeout {
        n280 = event-data() -> ()  [unwired: 1 in, 3 out]
      }
      event "Disable Vison After Auto": Mouse Enter; "Disable Vison After Auto": Mouse Leave {
        n281 = event-data() -> ("Type"=w473:T26)  [unwired: 1 in, 2 out]
        n282 = Equal?(x=w473, y=lveventtype."Mouse Enter") -> (x = y?=w471:bool)
        n283 = property on="Disable Vison After Auto" class="Bool (strict)"("Caption.Visible"=w471) -> ()  [unwired: 2 in, 2 out]
      }
      event "Use Hot Goal": Mouse Enter; "Use Hot Goal": Mouse Leave {
        n284 = event-data() -> ("Type"=w475:T26)  [unwired: 1 in, 3 out]
        n285 = Equal?(x=w475, y=lveventtype."Mouse Enter") -> (x = y?=w474:bool)
        n286 = property on="Use Hot Goal" class="Bool (strict)"("Caption.Visible"=w474) -> ()  [unwired: 2 in, 2 out]
      }
      event "Shoot During Auto": Mouse Enter; "Shoot During Auto": Mouse Leave {
        n287 = event-data() -> ("Type"=w478:T26)  [unwired: 1 in, 3 out]
        n288 = Equal?(x=w478, y=lveventtype."Mouse Enter") -> (x = y?=w477:bool)
        n289 = property on="Shoot During Auto" class="Bool (strict)"("Caption.Visible"=w477) -> ()  [unwired: 2 in, 2 out]
      }
      event "code too slow": Mouse Enter; "code too slow": Mouse Leave {
        n290 = event-data() -> ("Type"=w481:T26)  [unwired: 1 in, 3 out]
        n291 = Equal?(x=w481, y=lveventtype."Mouse Enter") -> (x = y?=w480:bool)
        n292 = property on="code too slow" class="Bool (strict)"("Caption.Visible"=w480) -> ()  [unwired: 2 in, 2 out]
      }
      event "Robot Found": Mouse Enter; "Robot Found": Mouse Leave {
        n293 = event-data() -> ("Type"=w484:T26)  [unwired: 1 in, 3 out]
        n294 = Equal?(x=w484, y=lveventtype."Mouse Enter") -> (x = y?=w483:bool)
        n295 = property on="Robot Found" class="Bool (strict)"("Caption.Visible"=w483) -> ()  [unwired: 2 in, 2 out]
      }
      event "Enable Full Driver Control": Mouse Enter; "Enable Full Driver Control": Mouse Leave {
        n296 = event-data() -> ("Type"=w487:T26)  [unwired: 1 in, 3 out]
        n297 = Equal?(x=w487, y=lveventtype."Mouse Enter") -> (x = y?=w486:bool)
        n298 = property on="Enable Full Driver Control" class="Bool (strict)"("Caption.Visible"=w486) -> ()  [unwired: 2 in, 2 out]
      }
    }
  }
  n299 = register-events(refnum<vi> refnum) -> (reference out=w15:refnum<event-registration>, error out=w14:errorcluster)  [unwired: 2 in]
  n300 = vi-ref "Playback Controls.vi"() -> (w16:refnum<vi>)
  n301 = call "Initialize Camera and CheckList.vi"("ListBox in"=w10) -> ("Cluster"=w18:cluster{"value":i32, "value":i32, "index":i32}, "Array"=w19:cluster{string[]}[], "File Refnum"=w17:T27)  [unwired: 8 in]
  n302 = property on="Camera Settings" class="Clust (strict)"("Val(Sgnl)"=w18) -> ()  [unwired: 2 in, 2 out]
  n303 = while {
    tunnel: w19 -> [w495]
    shift-right: [w494] -> _
    shift-left: w17 -> [w493]
    tunnel: [w492] -> _
    tunnel: w16 -> [w491]
    tunnel: w15 -> [w490]
    tunnel: w14 -> [_]
    tunnel: w9 -> [w489]
    i -> [w492]
    stop <- FALSE stop-if-true
    n304 = event shown="[0] Timeout" {
      selector: w490 -> [_ _ _ _ _ _]
      dyn-events: _ -> [_ _ _ _ _ _]
      timeout: u32 60 ("milliseconds to wait") -> [_ _ _ _ _ _]
      tunnel: w495 -> [_ _ _ w528 w558 _]
      tunnel: [w498 w502 w514 w527 w551 w563] -> w494
      tunnel: w493 -> [w498 w502 w514 w526 w551 w563]
      tunnel: w491 -> [_ _ _ _ _ w566]
      tunnel: w489 -> [_ _ _ _ _ _]
      event Timeout {
        n305 = event-data() -> ()  [unwired: 1 in, 1 out]
        n306 = case shown="\"Network Variables\"" "Dashboard Tab" {
          tunnel: [_ w501] -> _
          frame "Debug System", Default {
          }
          frame "Network Variables" {
            n307 = control-ref of="Tree"() -> (w500:refnum<vi>)
            n308 = call <vilib>:"NT Read and Format Entries as Tree.vi"("Tree Refnum"=w500) -> ("Formatted Strings"=w501:cluster{"Name":string, "Value":string}[])  [unwired: 9 in, 1 out]
          }
        }
      }
      event "Listbox": Double Click {
        n309 = event-data() -> ("PlatMods.Shift"=w503:bool, "Row"=w505:i32)  [unwired: 1 in]
        n310 = case shown="True" w503 {
          tunnel: w505 -> [w509 _]
          tunnel: 1 -> [w508 _]
          frame False {
            n311 = property on="Listbox" class="LstBox (strict)"() -> ("Item Symbols"=w507:i32[])  [unwired: 2 in, 2 out]
            n312 = Replace Array Subset(array=w507, new element=w508, index=w509) -> (w506:i32[])
            n313 = property on="Listbox" class="LstBox (strict)"("Item Symbols"=w506) -> ()  [unwired: 2 in, 2 out]
          }
          frame True {
            w510 = 0 ("Top Row")
            n314 = property on="Listbox" class="LstBox (strict)"() -> ("Number of Rows"=w512:u32)  [unwired: 2 in, 2 out]
            n315 = Initialize Array(0, w512) -> (w511:i32[])
            n316 = property on="Listbox" class="LstBox (strict)"("Top Row"=w510, "Value"=w510, "Item Symbols"=w511) -> ()  [unwired: 2 in, 2 out]
          }
        }
      }
      event "Listbox": Key Down {
        n317 = event-data() -> ("VKey"=w516:T28)  [unwired: 1 in]
        n318 = case shown="\"Left\", \"Right\"" w516 {
          selector: w516 -> [w521 _]
          tunnel: eventvkey."Left" ("VKey") -> [w519 _]
          frame "Left", "Right" {
            n319 = Equal?(x=w519, y=w521) -> (x = y?=w520:bool)
            n320 = Select(t=0, s=w520, f=1) -> (s? t:f=w522:i32)
            n321 = property on="Listbox" class="LstBox (strict)"() -> ("Item Symbols"=w525:i32[])  [unwired: 2 in, 2 out]
            n322 = Replace Array Subset(array=w525, new element=w522, index="Listbox") -> (w524:i32[])
            n323 = property on="Listbox" class="LstBox (strict)"("Item Symbols"=w524) -> ()  [unwired: 2 in, 2 out]
          }
          frame Default {
          }
        }
      }
      event "DB Camera Config": Value Change {
        n324 = event-data() -> ("NewVal"=w529:bool)  [unwired: 1 in]
        n325 = case shown="False" w529 {
          tunnel: w528 -> [w538 _]
          tunnel: [w531 w549] -> w527
          tunnel: w526 -> [w530 w549]
          frame False {
            w545 = "Camera"
            w548 = FALSE ("Visible")
            n326 = local read "Camera Settings"() -> (w537:T5)
            n327 = Index Array(array=w538) -> (element=w541:cluster{string[]})  [unwired: 1 in]
            n328 = Unbundle(w537) -> ("Frame Rate"=w536:i32, "Compression"=w535:i32, "Size"=w539:u16)
            n329 = Unbundle(w541) -> (w540:string[])
            n330 = Index Array(array=w540, index=w539) -> (element=w534:string)
            n331 = call-poly <vilib>:"Write Key.vi"("section"=w545, "value"=w534, "key"="Size", "refnum"=w530) -> ("refnum out"=w547:T27)  [unwired: 2 in, 5 out]
            n332 = call-poly <vilib>:"Write Key.vi"("section"=w545, "value"=w536, "key"="FrameRate", "refnum"=w547) -> ("refnum out"=w546:T27)  [unwired: 1 in, 6 out]
            n333 = property on="Camera Settings" class="Clust (strict)"("Visible"=w548) -> ()  [unwired: 2 in, 2 out]
            n334 = local write "DB Camera Config"(w548) -> ()
            n335 = call-poly <vilib>:"Write Key.vi"("section"=w545, "value"=w535, "key"="Compression", "refnum"=w546) -> ("refnum out"=w532:T27)  [unwired: 1 in, 6 out]
            n336 = call <vilib>:"Close Config Data.vi"("refnum"=w532) -> ("file path"=w533:path)  [unwired: 2 in, 8 out]
            n337 = call <vilib>:"Open Config Data.vi"("configuration file path"=w533) -> ("refnum"=w531:T27)  [unwired: 8 in, 2 out]
          }
          frame True {
            n338 = property on="Camera Settings" class="Clust (strict)"("Visible"=TRUE) -> ()  [unwired: 2 in, 2 out]
          }
        }
      }
      event "Camera Settings": Value Change {
        n339 = event-data() -> ("NewVal"=w562:T5)  [unwired: 1 in]
        n340 = Index Array(array=w558) -> (element=w557:cluster{string[]})  [unwired: 1 in]
        n341 = Unbundle(w562) -> ("Frame Rate"=w553:i32, "Compression"=w552:i32, "Size"=w555:u16)
        n342 = Unbundle(w557) -> (w556:string[])
        n343 = Index Array(array=w556, index=w555) -> (element=w554:string)
        n344 = Format Into String(format string="%s   %dfps   %d%%", w554, w553, w552) -> (resulting string=w559:string)  [unwired: 2 in, 1 out]
        n345 = Build Array(w559) -> (w560:string[])
        n346 = property on="DB Camera Config" class="Bool (strict)"("Strings [4]"=w560) -> ()  [unwired: 2 in, 2 out]
      }
      event Panel Close {
        # "Abort playback window and ourself"
        n347 = event-data() -> ()  [unwired: 1 in, 4 out]
        n348 = invoke class="VI" method="FP.Close"(reference=w566) -> (reference out=w565:refnum<vi>)  [unwired: 2 in, 2 out]
        n349 = invoke class="VI" method="Abort VI"(reference=w565) -> (error out=w564:errorcluster)  [unwired: 2 in, 2 out]
        n350 = invoke class="VI" method="Abort VI"(error in=w564) -> ()  [unwired: 2 in, 3 out]
      }
    }
  }
  n351 = property on="Camera Settings" class="Clust (strict)"("Visible"=w21) -> ()  [unwired: 2 in, 2 out]
  n352 = local write "DB Camera Config"(w21) -> ()
